vi "svm_add_model_padding.vi"(8 "error in (no error)":errorcluster, 11 "Model":T1) -> (0 "error out":errorcluster, 3 "Padded model":T6)   [LabVIEW 2015]
uses:
  Controls/svm_model_padded.ctl
  Controls/svm_parameter.ctl
  Controls/svm_type.ctl
  Controls/svm_kernel_type.ctl
  Controls/svm_node_padded.ctl
  Controls/svm_model.ctl
  Controls/svm_node.ctl
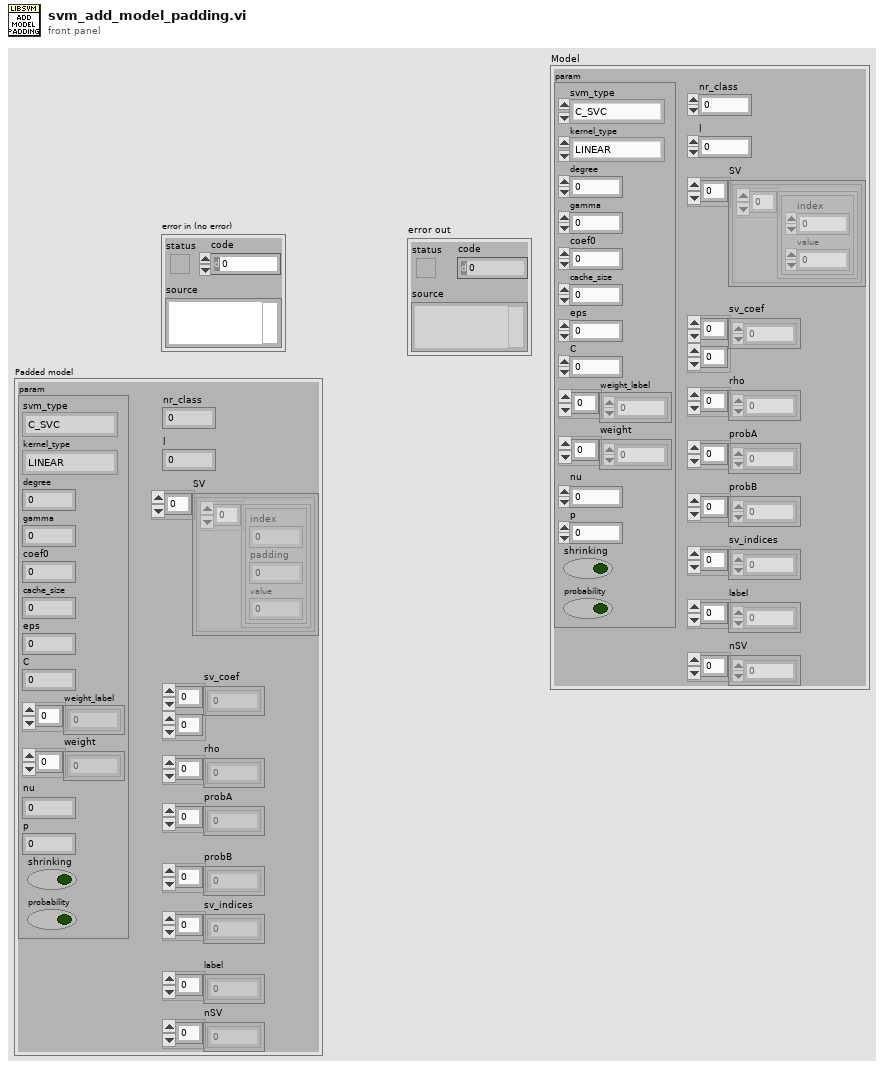
[diagram p1: front panel]
types:
  T1 = typedef "svm_model.ctl" = cluster{"param":T2, "nr_class":i32, "l":i32, "SV":cluster{"Array":T5[]}[], "sv_coef":dbl[][], "rho":dbl[], "probA":dbl[], "probB":dbl[], "sv_indices":i32[], "label":i32[], "nSV":i32[]}
  T2 = typedef "svm_parameter.ctl" = cluster{"svm_type":T3, "kernel_type":T4, "degree":i32, "gamma":dbl, "coef0":dbl, "cache_size":dbl, "eps":dbl, "C":dbl, "weight_label":i32[], "weight":dbl[], "nu":dbl, "p":dbl, "shrinking":bool, "probability":bool}
  T3 = typedef "svm_type.ctl" = enum32{"C_SVC", "NU_SVC", "ONE_CLASS", "EPSILON_SVR", "NU_SVR"}
  T4 = typedef "svm_kernel_type.ctl" = enum32{"LINEAR", "POLY", "RBF", "SIGMOID", "PRECOMPUTED"}
  T5 = typedef "svm_node.ctl" = cluster{"index":i32, "value":dbl}
  T6 = typedef "svm_model_padded.ctl" = cluster{"param":T2, "nr_class":i32, "l":i32, "SV":cluster{"Array":T7[]}[], "sv_coef":dbl[][], "rho":dbl[], "probA":dbl[], "probB":dbl[], "sv_indices":i32[], "label":i32[], "nSV":i32[]}
  T7 = typedef "svm_node_padded.ctl" = cluster{"index":i32, "padding":i32, "value":dbl}
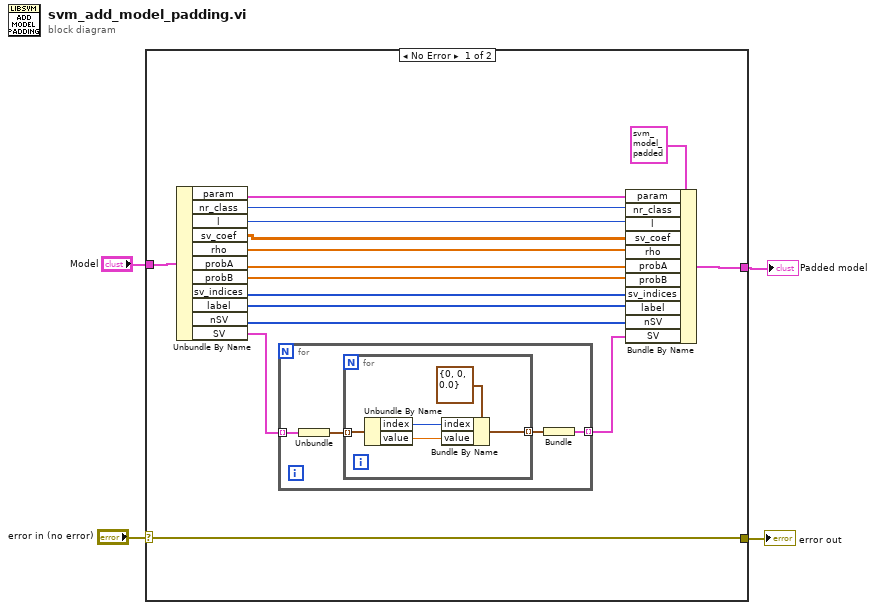
[diagram p0: block diagram]
diagram:
  n1 = case shown="No Error" "error in (no error)" {
    selector: "error in (no error)" -> [w8 w30]
    tunnel: [w8 w30] -> w4
    tunnel: "Model" -> [w20 _]
    tunnel: [w19 _] -> w1
    frame No Error {
      n2 = Unbundle By Name(w20) -> ("param"=w18:T2, "nr_class"=w17:i32, "l"=w16:i32, "sv_coef"=w15:dbl[][], "rho"=w14:dbl[], "probA"=w13:dbl[], "probB"=w12:dbl[], "sv_indices"=w11:i32[], "label"=w10:i32[], "nSV"=w9:i32[], "SV"=w7:cluster{"Array":T5[]}[])
      n3 = for {
        tunnel: w7 -> [w24] mode=indexing
        tunnel: [w21] -> w6 mode=indexing
        n4 = Unbundle(w24) -> ("Array"=w23:T5[])
        n5 = for {
          tunnel: w23 -> [w29] mode=indexing
          tunnel: [w26] -> w22 mode=indexing
          n6 = Unbundle By Name(w29) -> ("index"=w28:i32, "value"=w27:dbl)
          n7 = Bundle By Name(cluster=T7 {"index"=0, "padding"=0, "value"=0.0} ("svm_node"), "index"=w28, "value"=w27) -> (w26:T7)
        }
        n8 = Bundle(w22) -> (w21:cluster{T7[]})  [unwired: 1 in]
      }
      n9 = Bundle By Name(cluster=T6 {"param"={"svm_type"=enum."C_SVC", "kernel_type"=enum."LINEAR", "degree"=0, "gamma"=0.0, "coef0"=0.0, "cache_size"=0.0, "eps"=0.0, "C"=0.0, "weight_label"=[], "weight"=[], "nu"=0.0, "p"=0.0, "shrinking"=FALSE, "probability"=FALSE}, "nr_class"=0, "l"=0, "SV"=[], "sv_coef"=[], "rho"=[], "probA"=[], "probB"=[], "sv_indices"=[], "label"=[], "nSV"=[]} ("svm_model"), "param"=w18, "nr_class"=w17, "l"=w16, "sv_coef"=w15, "rho"=w14, "probA"=w13, "probB"=w12, "sv_indices"=w11, "label"=w10, "nSV"=w9, "SV"=w6) -> (w19:T6)
    }
    frame Error {
    }
  }
  "error out" <- w4
  "Padded model" <- w1
